vi "Create and Add Instruments.vi"(7 "Is Target?":bool, 8 "Error In":errorcluster, 10 "Physical Intr CFGs":string[](array[string]), 11 "MSS in":refnum<class "Measure and Stimulus Subsystems.lvclass">) -> (0 "Error Out":errorcluster, 1 "Target Physical Instr CFGs":string[](array[string]), 3 "MSS out":refnum<class "Measure and Stimulus Subsystems.lvclass">)   [LabVIEW 2023, in "HAL GOOP4.lvlib" / "Measure and Stimulus Subsystems.lvclass"]
uses:
  Measure and Stimulus Subsystems.lvclass
  CFG Target/CFG Target.lvclass
  Configuration/Configuration JSON/Configuration JSON Base/CFG JSON.lvclass
  <vilib>/JDP Science/JSONtext/Find Item.vi
  <vilib>/JDP Science/JSONtext/Next JSON Value.vi
  <vilib>/JDP Science/JSONtext/String Subset.vi
  <vilib>/JDP Science/JSONtext/Parsing/Advance past next JSON Value (inlined COPY).vi
  <vilib>/JDP Science/JSONtext/Parsing/Advance past whitespace.vi
  <vilib>/JDP Science/JSONtext/Parsing/Advance past String.vi
  <vilib>/JDP Science/JSONtext/Parsing/Advance past Number.vi
  <vilib>/JDP Science/JSONtext/Parsing/Advance past Line Ending.vi
  <vilib>/JDP Science/JSONtext/Parsing/Parse Full Path or Item Name.vi
  <vilib>/JDP Science/JSONtext/Parsing/Advance past Array.vi
  <vilib>/JDP Science/JSONtext/Parsing/Advance past Object.vi
  <vilib>/JDP Science/JSONtext/support/Error Cluster From Code.vi
  <vilib>/JDP Science/JSONtext/Offset/Find Item Locations by Path.vi
  <vilib>/JDP Science/JSONtext/JSON text to Variant.vi
  <vilib>/JDP Science/JSONtext/LVClass Serializer/JSONtext LVClass Serializer.lvclass
  Measure and Stimulus Subsystems.lvclass/Measure and Stimulus Subsystems.ctl
  Instrument/Instrument.lvclass
  25b25780-789a-4bec-9ea7-0fafa89e9659.vi
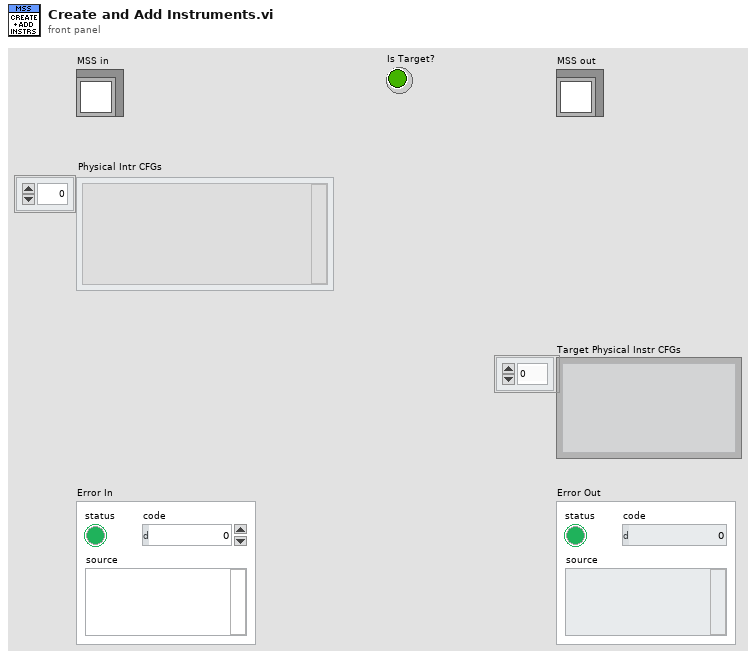
[diagram p1: front panel]
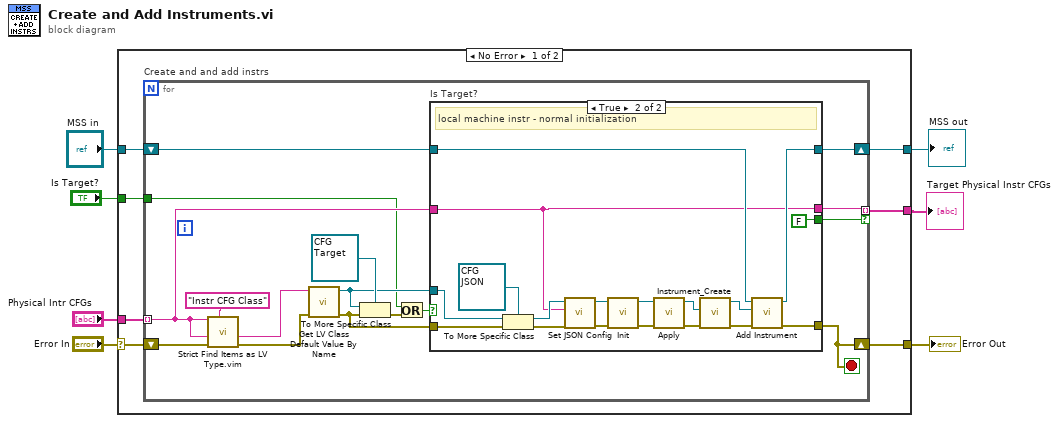
[diagram p0: block diagram]
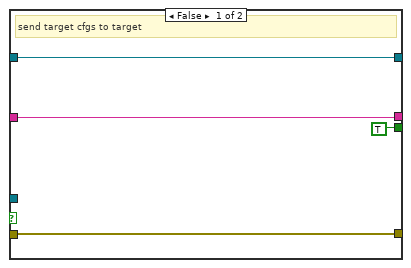
[diagram p2: hidden frame]
diagram:
  n1 = case shown="No Error" "Error In" {
    selector: "Error In" -> [w12 w53]
    tunnel: [w10 w53] -> w7
    tunnel: [w13 w54] -> w3
    tunnel: "MSS in" -> [w14 w54]
    tunnel: "Physical Intr CFGs" -> [w11 _]
    tunnel: [w9 _] -> w2
    tunnel: "Is Target?" -> [w8 _]
    frame No Error {
      n2 = for "Create and and add instrs" {
        shift-right: [w21] -> w10
        shift-left: w12 -> [w28]
        tunnel: w11 -> [w23] mode=indexing
        shift-right: [w27] -> w13
        shift-left: w14 -> [w24]
        tunnel: [w22] -> w9 mode=indexing if=w19
        tunnel: w8 -> [w16]
        stop <- w21 stop-if-true
        n3 = call "Strict Find Items as LV Type.vim"("$Path or Item Name"="Instr CFG Class", "error in"=w28, "Data Type and Default Value"=w23, "JSON"=w23) -> ("error out"=w15:errorcluster, "Data out"=w20:string)  [unwired: 6 in]
        n4 = call <vilib>:"Get LV Class Default Value By Name.vi"("error in (no error)"=w15, "class name"=w20) -> ("error out"=w26:errorcluster, "object"=w25:refnum<class>)  [unwired: 8 in]
        n5 = To More Specific Class(target class=refnum<class "CFG Target.lvclass"> refnum ("CFG Target.lvclass"), reference=w25, error in=w26) -> (error out=w17:errorcluster)  [unwired: 1 out]
        n6 = Or(x=w16, y=w17) -> (x .or. y?=w18:bool)
        n7 = case "Is Target?" shown="True" w18 {
          tunnel: [w33 w41] -> w21
          tunnel: w24 -> [w34 w40]
          tunnel: [w34 w39] -> w27
          tunnel: w26 -> [w33 w38]
          tunnel: w25 -> [_ w37]
          tunnel: w23 -> [w32 w36]
          tunnel: [w32 w36] -> w22
          tunnel: [TRUE FALSE] -> w19
          frame False {
            # "send target cfgs to target"
          }
          frame True {
            # "local machine instr - normal initialization"
            n8 = To More Specific Class(target class=refnum<class "CFG JSON.lvclass"> refnum ("HAL GOOP4.lvlib:CFG JSON Base.lvclass"), reference=w37, error in=w38) -> (specific class reference=w49:refnum<class "CFG JSON.lvclass">, error out=w48:errorcluster)
            n9 = call "Set JSON Config.vi"("error in (no error)"=w48, "<JSON>Config>"=w36, "CFG Base in"=w49) -> ("error out"=w51:errorcluster, "CFG Base out"=w46:refnum<class "CFG JSON.lvclass">)  [unwired: 7 in]
            n10 = call-dynamic "Init.vi"("error in (no error)"=w51, "IConfigure in"=w46) -> ("error out"=w47:errorcluster, "IConfigure out"=w44:refnum<class "CFG JSON.lvclass">)  [unwired: 8 in]
            n11 = call-dynamic "Apply.vi"("error in (no error)"=w47, "IConfigure in"=w44) -> ("error out"=w45:errorcluster, "IConfigure out"=w43:refnum<class "CFG JSON.lvclass">)  [unwired: 8 in]
            n12 = call "Instrument_Create.vi"("Error In"=w45, "IConfigure"=w43) -> ("Error Out"=w52:errorcluster, "reference out"=w42:refnum<class "Instrument.lvclass">)  [unwired: 8 in]
            n13 = call "Add Instrument.vi"("error in"=w52, "Instrument"=w42, "MSS in"=w40) -> ("error out"=w41:errorcluster, "MSS out"=w39:refnum<class "Measure and Stimulus Subsystems.lvclass">)  [unwired: 7 in]
          }
        }
      }
    }
    frame Error {
    }
  }
  "MSS out" <- w3
  "Error Out" <- w7
  "Target Physical Instr CFGs" <- w2
